vi "rotation.vi"(7 "On/Off\nRight/Left":bool, 8 "error in (no error)":errorcluster) -> (0 "error out":errorcluster, 3 "angle Z":ext)   [LabVIEW 2017]
uses:
  <vilib>/myRIO/Instrument Drivers/Onboard IO/I2C/typedefs/I2C Reference.ctl
  <vilib>/myRIO/Common/Instrument Driver Framework/Utilities/typedefs/myRIO Generic Hardware Reference.ctl
  <vilib>/myRIO/Common/Instrument Driver Framework/Utilities/typedefs/Hardware Version Enum.ctl
  <vilib>/myRIO/Common/Instrument Driver Framework/Utilities/typedefs/myRIO v1.0 Reference.ctl
  <vilib>/myRIO/Common/Instrument Driver Framework/Utilities/typedefs/Generic FPGA Reference.ctl
  <vilib>/myRIO/Common/Instrument Driver Framework/myRIO v1.0/I2C/typedefs/I2C Channels Enum.ctl
  <vilib>/myRIO/Instrument Drivers/Onboard IO/I2C/typedefs/I2C Configuration.ctl
  <vilib>/myRIO/Instrument Drivers/Onboard IO/I2C/typedefs/I2C Transfer Rate.ctl
  <vilib>/userdefined/High Color/nirio_resource_hc.ctl
  <vilib>/myRIO/Common/Instrument Driver Framework/myRIO v1.0/Encoder/typedefs/Encoder Signal Mode.ctl
  <vilib>/myRIO/Instrument Drivers/Onboard IO/Encoder/typedefs/Encoder Reference.ctl
  <vilib>/myRIO/Common/Instrument Driver Framework/myRIO v1.0/Encoder/typedefs/Encoder Channels Enum.ctl
  <vilib>/myRIO/Common/Instrument Driver Framework/myRIO v1.0/Encoder/typedefs/Encoder Configuration v1.0.ctl
  <vilib>/myRIO/Common/Instrument Driver Framework/myRIO v1.0/I2C/vis/myRIO v1.1 Open I2C.vi
  <vilib>/myRIO/Common/Instrument Driver Framework/Utilities/vis/Is FPGA Ref Available.vi
  <vilib>/myRIO/Common/Instrument Driver Framework/myRIO v1.0/Encoder/vis/myRIO v1.1 Open Encoder.vi
  <vilib>/myRIO/Instrument Drivers/Onboard IO/Encoder/vis/Read.vi
  <vilib>/myRIO/Common/Instrument Driver Framework/Utilities/vis/Validate Channels.vi
  <vilib>/myRIO/Common/Instrument Driver Framework/myRIO v1.0/I2C/vis/myRIO v1.0 Reserve I2C.vi
  <vilib>/myRIO/Common/Instrument Driver Framework/myRIO v1.0/Encoder/vis/myRIO v1.0 Reserve Encoder.vi
  <vilib>/myRIO/Common/Instrument Driver Framework/myRIO v1.0/I2C/vis/myRIO v1.0 Close I2C.vi
  <vilib>/myRIO/Common/Instrument Driver Framework/myRIO v1.0/I2C/vis/myRIO v1.0 Build MUX Configuration I2C.vi
  <vilib>/myRIO/Common/Instrument Driver Framework/myRIO v1.0/Resource Manager/vis/myRIO v1.0 Reserve Channel List.vi
  <vilib>/myRIO/Common/Instrument Driver Framework/myRIO v1.0/Encoder/vis/myRIO v1.0 Build MUX Configuration Encoder.vi
  <vilib>/myRIO/Common/Instrument Driver Framework/myRIO v1.0/I2C/vis/myRIO v1.0 Unreserve I2C.vi
  <vilib>/myRIO/Common/Instrument Driver Framework/myRIO v1.0/Resource Manager/vis/myRIO v1.0 Create Configuration List.vi
  <vilib>/myRIO/Common/Instrument Driver Framework/myRIO v1.0/Resource Manager/vis/myRIO v1.0 Reserve Channel.vi
  <vilib>/myRIO/Common/Instrument Driver Framework/myRIO v1.0/Resource Manager/vis/myRIO v1.0 Unreserve Channel.vi
  <vilib>/myRIO/Common/Instrument Driver Framework/myRIO v1.0/Resource Manager/vis/myRIO v1.0 Unreserve Channel List.vi
  <vilib>/myRIO/Common/Instrument Driver Framework/myRIO v1.0/Resource Manager/vis/myRIO v1.0 Build Mutex Name.vi
  <vilib>/Utility/VariantDataType/GetNumericInfo.vi
  <vilib>/Utility/error.llb/Error Cluster From Error Code.vi
  <vilib>/myRIO/Common/Instrument Driver Framework/myRIO v1.0/myRIO v1.1 Open.vi
  <vilib>/myRIO/Common/Instrument Driver Framework/Utilities/vis/IO Manager.vi
  <vilib>/myRIO/Common/Instrument Driver Framework/Utilities/vis/Configuration Manager.vi
  <vilib>/myRIO/Common/Instrument Driver Framework/myRIO v1.0/Resource Manager/vis/myRIO v1.0 Configure IO.vi
  <vilib>/myRIO/Common/Instrument Driver Framework/myRIO v1.0/myRIO v1.0 Close.vi
  <vilib>/imath/engines/lvmath2/RunTimeEngine/Managers/WorkSpace/UID Generator.vi
  <vilib>/imath/engines/lvmath2/RunTimeEngine/RunTimeType/NIMS_RunTimeType_From StrictType (excl LVString).vi
  <instcachedir>/0/NIMS_RunTimeType_From StrictType (excl LVString)_1019F277F0A747EDBCA0F6C52CA54500.lvgen/NIMS_RunTimeType_From StrictType (excl LVString)_1019F277F0A747EDBCA0F6C52CA54500_000.vi
  <vilib>/imath/engines/lvmath2/RunTimeEngine/LocalVariableDefStatement/MC_LocalVariableDefStatement_Display.vi
  <vilib>/imath/engines/lvmath2/RunTimeEngine/Managers/SymbolTable/Clear UID.vi
  <vilib>/imath/engines/lvmath2/RunTimeEngine/NodeEndStatement/NIMS_NodeEndStatement_Output.vi
  <instcachedir>/0/NIMS_NodeEndStatement_Output_53EC0D466D134D7ABD903AC30B43404B.lvgen/NIMS_NodeEndStatement_Output_53EC0D466D134D7ABD903AC30B43404B_013.vi
  <vilib>/imath/engines/lvmath2/RunTimeEngine/ErrorHandling/NIMS_Finalize Error.vi
  <vilib>/myRIO/Common/Instrument Driver Framework/myRIO v1.0/Encoder/vis/myRIO v1.0 Configure Encoder.vi
  <vilib>/myRIO/Common/Instrument Driver Framework/myRIO v1.0/Encoder/vis/myRIO v1.0 Read Encoder.vi
  <vilib>/myRIO/Common/Instrument Driver Framework/myRIO v1.0/I2C/vis/myRIO v1.0 Shutdown I2C.vi
  <vilib>/myRIO/Instrument Drivers/Onboard IO/I2C/vis/myRIO I2C Open.xnode
  <vilib>/myRIO/Express VI/Onboard IO/Encoder/Encoder Express VI.xnode
  <vilib>/myRIO/Instrument Drivers/Onboard IO/Encoder/vis/myRIO Encoder Open.xnode
  <vilib>/myRIO/Common/Instrument Driver Framework/myRIO v1.0/Encoder/typedefs/Encoder Count Direction Enum.ctl
  <vilib>/imath/engines/lvmath2/RunTimeEngine/Managers/SymbolTable/NIMS_WorkSpace.lvlib
  <vilib>/myRIO/Instrument Drivers/Onboard IO/Encoder/Encoder.lvlib
  <vilib>/myRIO/Instrument Drivers/Onboard IO/I2C/I2C.lvlib
panel:
  out "rotate to":ext
  in  "Stop Motor(false block)":bool
  in  "Stop Motor(true block)":bool
  in  "Stop Button":bool
  out "zMax right":ext
  out "zMin right":ext
  out "zMin left":ext
  out "zMax left":ext
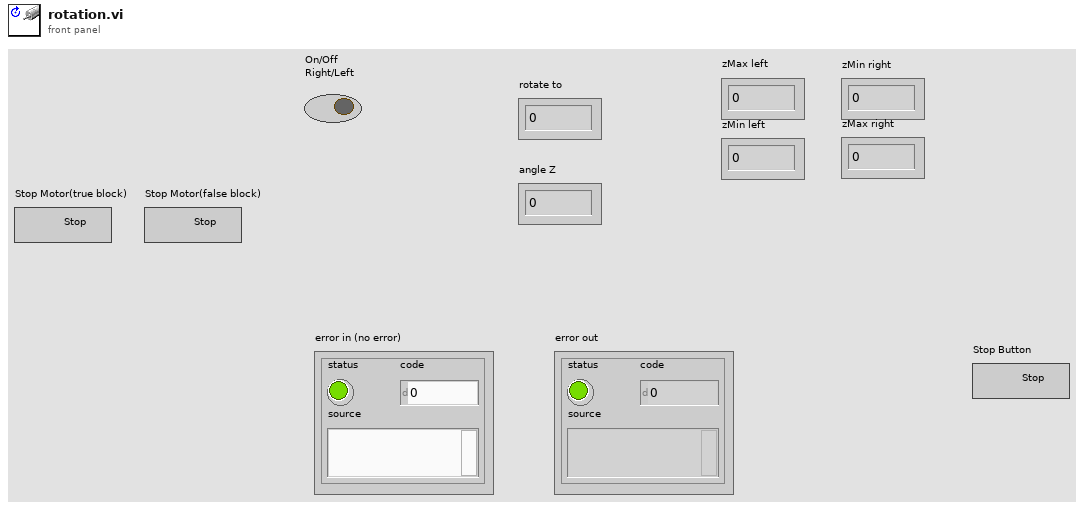
[diagram p1: front panel]
types:
  T1 = typedef "I2C.lvlib/I2C Reference.ctl" = cluster{"myRIO Reference":T2, "I2C Channels Enum":T6, "I2C Configuration":T7}
  T2 = typedef "myRIO Generic Hardware Reference.ctl" = cluster{"myRIO Model":T3, "myRIO Hardware Reference":T4}
  T3 = typedef "Hardware Version Enum.ctl" = enum16{"Unknown", "myRIO-1900", "myRIO-1950", "roboRIO", "NI ELVIS RIO CM"}
  T4 = typedef "myRIO v1.0 Reference.ctl" = cluster{"Generic FPGA Reference":T5, "Allow multiple opens":bool}
  T5 = typedef "Generic FPGA Reference.ctl" = refnum<k20>
  T6 = typedef "I2C Channels Enum.ctl" = enum16{"Not Connected", "A/I2C", "B/I2C", "I2C/I2C"}
  T7 = typedef "I2C.lvlib/I2C Configuration.ctl" = cluster{"I2C Transfer Rate":T8}
  T8 = typedef "I2C.lvlib/I2C Transfer Rate.ctl" = enum16{"Standard mode (100 kbps)", "Fast mode (400 kbps)"}
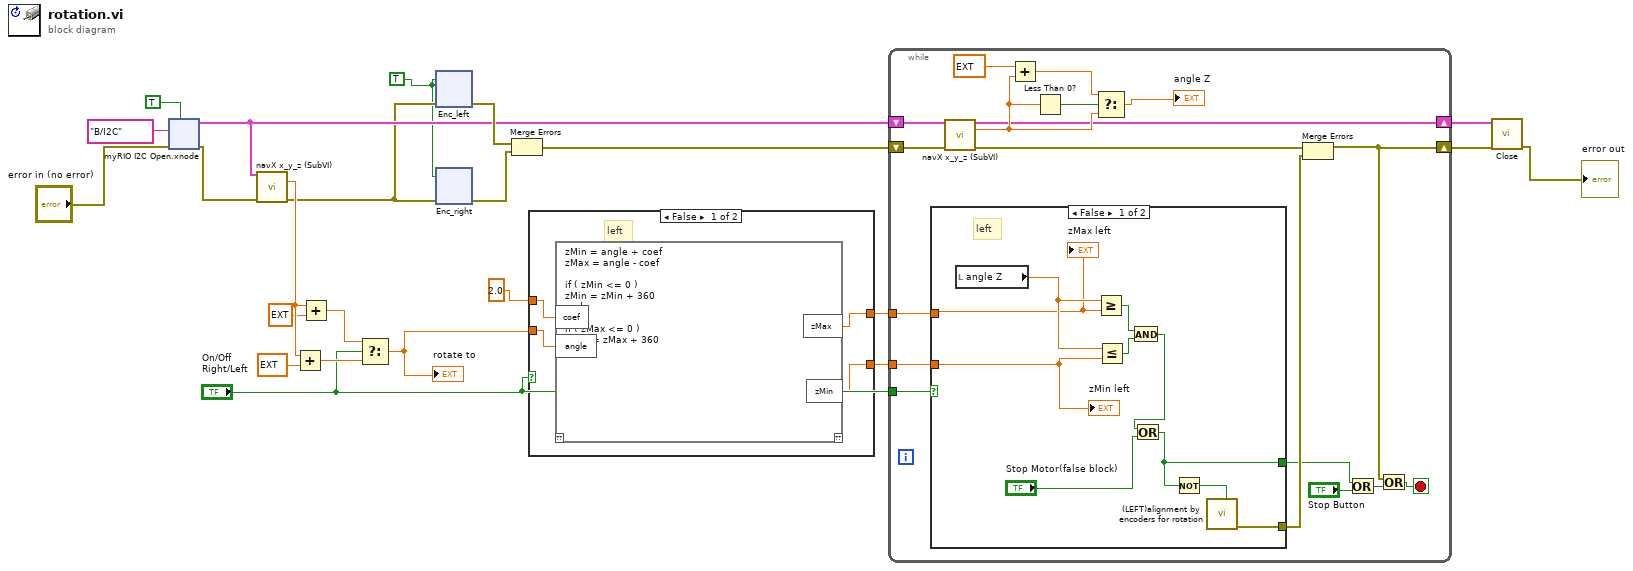
[diagram p0: block diagram]
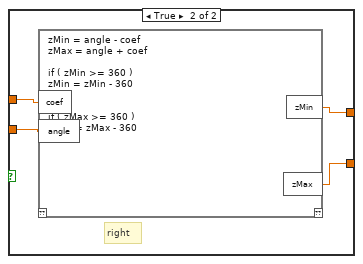
[diagram p2: hidden frame]
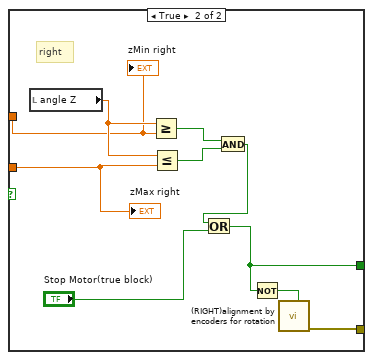
[diagram p3: hidden frame]
diagram:
  w1 = TRUE
  n1 = xnode "myRIO I2C Open.xnode"("error in (no error)"="error in (no error)", "Allow multiple opens?"=TRUE, "Channel Name"=tag "B/I2C") -> ("error out"=w3:errorcluster, "I2C Ref Out"=w16:T1)
  n2 = call "navX x_y_z (SubVI).vi"("I2C Ref Out in"=w16, "error in (no error)"=w3) -> ("value Z"=w13:ext, "error out"=w9:errorcluster)  [unwired: 9 in, 3 out]
  n3 = Add(x=w13, y=ext -90.0) -> (x+y=w15:ext)
  n4 = Add(x=w13, y=ext 90.0) -> (x+y=w14:ext)
  n5 = Select(t=w14, s="On/Off\nRight/Left", f=w15) -> (s? t:f=w6:ext)
  "rotate to" <- w6
  n6 = xnode "Enc_left"("error in (no error)"=w9, "Reset Counter"=w1) -> ("error out"=w18:errorcluster)  [unwired: 3 out]
  n7 = xnode "Enc_right"("error in (no error)"=w9, "Reset Counter"=w1) -> ("error out"=w17:errorcluster)  [unwired: 3 out]
  n8 = Merge Errors(w18, w17) -> (w23:errorcluster)
  n9 = case shown="False" "On/Off\nRight/Left" {
    tunnel: 2.0 ("coef") -> [w27 w144]
    tunnel: w6 -> [w26 w143]
    tunnel: [w24 w142] -> w5
    tunnel: [w25 w141] -> w4
    frame False {
      # "left"
      n10 = mathscript code="zMin = angle + coef\nzMax = angle - coef\n\nif ( zMin <= 0 )\nzMin = zMin + 360\nend\n\nif ( zMax <= 0 )\nzMax = zMax + 360\nend"("angle"=w26, "coef"=w27) -> ("zMin"=w25:ext, "zMax"=w24:ext)  [unwired: 1 in, 1 out]
    }
    frame True {
      # "right"
      n11 = mathscript code="zMin = angle - coef\nzMax = angle + coef\n\nif ( zMin >= 360 )\nzMin = zMin - 360\nend\n\nif ( zMax >= 360 )\nzMax = zMax - 360\nend"("angle"=w143, "coef"=w144) -> ("zMin"=w142:ext, "zMax"=w141:ext)  [unwired: 1 in, 1 out]
    }
  }
  n12 = while {
    shift-right: [w258] -> w22
    shift-left: w23 -> [w273]
    tunnel: "On/Off\nRight/Left" -> [w267]
    shift-right: [w266] -> w19
    shift-left: w16 -> [w274]
    tunnel: w5 -> [w262]
    tunnel: w4 -> [w261]
    stop <- w259 stop-if-true
    n13 = case shown="False" w267 {
      tunnel: [w278 w289] -> w263
      tunnel: [w282 w287] -> w269
      tunnel: w262 -> [w277 w286]
      tunnel: w261 -> [w276 w288]
      frame False {
        # "left"
        n14 = local read "angle Z"() -> (w283:ext)
        n15 = Greater Or Equal?(x=w283, y=w277) -> (x >= y?=w284:bool)
        n16 = Less Or Equal?(x=w283, y=w276) -> (x <= y?=w285:bool)
        n17 = And(x=w284, y=w285) -> (x .and. y?=w281:bool)
        n18 = Or(x=w281, y="Stop Motor(false block)") -> (x .or. y?=w278:bool)
        n19 = Not(x=w278) -> (.not. x?=w279:bool)
        n20 = call "(LEFT)alignment by encoders for rotation.vi"("On/Off"=w279) -> ("error out"=w282:errorcluster)  [unwired: 10 in]
        "zMin left" <- w276
        "zMax left" <- w277
      }
      frame True {
        # "right"
        n21 = local read "angle Z"() -> (w293:ext)
        n22 = Greater Or Equal?(x=w293, y=w286) -> (x >= y?=w295:bool)
        n23 = Less Or Equal?(x=w293, y=w288) -> (x <= y?=w294:bool)
        n24 = And(x=w295, y=w294) -> (x .and. y?=w292:bool)
        n25 = Or(x=w292, y="Stop Motor(true block)") -> (x .or. y?=w289:bool)
        n26 = Not(x=w289) -> (.not. x?=w290:bool)
        n27 = call "(RIGHT)alignment by encoders for rotation.vi"("On/Off"=w290) -> ("error out"=w287:errorcluster)  [unwired: 10 in]
        "zMax right" <- w288
        "zMin right" <- w286
      }
    }
    n28 = call "navX x_y_z (SubVI).vi"("I2C Ref Out in"=w274, "error in (no error)"=w273) -> ("I2C Ref Out out"=w266:T1, "value Z"=w271:ext, "error out"=w268:errorcluster)  [unwired: 9 in, 2 out]
    n29 = Add(x=ext 360.0, y=w271) -> (x+y=w270:ext)
    n30 = Less Than 0?(x=w271) -> (x < 0?=w272:bool)
    n31 = Select(t=w270, s=w272, f=w271) -> (s? t:f=→"angle Z":ext)
    n32 = Merge Errors(w268, w269) -> (w258:errorcluster)
    n33 = Or(x=w263, y="Stop Button") -> (x .or. y?=w260:bool)
    n34 = Or(x=w258, y=w260) -> (x .or. y?=w259:bool)
  }
  n35 = call <vilib>:"Close.vi"("error in (no error)"=w22, "I2C Ref In"=w19) -> ("error out"=→"error out":errorcluster)  [unwired: 9 in]
